vi "Send Temperature Status.vi"(8 "error in (no error)":errorcluster, 11 "Stream in":refnum<class "Stream.lvclass">) -> (0 "error out":errorcluster, 3 "Stream out":refnum<class "Stream.lvclass">)   [LabVIEW 2018, in "Stream.lvclass"]
uses:
  Stream.lvclass
  Stream.lvclass/Stream.ctl
  Interface/Interface.lvclass/Interface.ctl
  Interface/Interface.lvclass
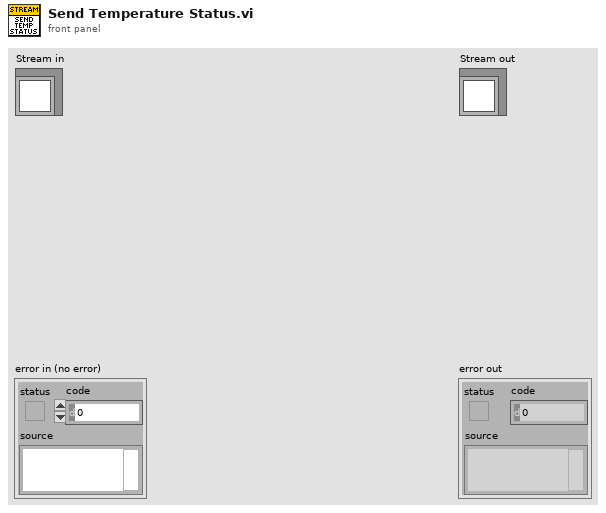
[diagram p1: front panel]
types:
  T1 = cluster{"Current Temperature":i16, "Temperatue Status":string}
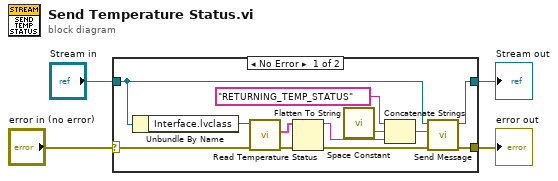
[diagram p0: block diagram]
diagram:
  n1 = case shown="No Error" "error in (no error)" {
    selector: "error in (no error)" -> [w7 w18]
    tunnel: [w16 w18] -> w2
    tunnel: [w14 w17] -> w1
    tunnel: "Stream in" -> [w15 w17]
    frame No Error {
      n2 = Unbundle By Name(w15) -> ("Interface.lvclass"=w6:refnum<class "Interface.lvclass">)
      n3 = call "Read Temperature Status.vi"("error in (no error)"=w7, "Interface in"=w6) -> ("error out"=w8:errorcluster, "Temperature Status"=w5:T1)  [unwired: 7 in, 1 out]
      n4 = Flatten To String(anything=w5, error in (no error)=w8) -> (data string=w10:string, error out=w13:errorcluster)  [unwired: 2 in, 1 out]
      n5 = call <vilib>:"Space Constant.vi"() -> ("String"=w11:string)
      n6 = Concatenate Strings("RETURNING_TEMP_STATUS", w11, w10) -> (w9:string)
      n7 = call "Send Message.vi"("error in (no error)"=w13, "Message"=w9, "Stream in"=w15) -> ("error out"=w16:errorcluster, "Stream out"=w14:refnum<class "Stream.lvclass">)  [unwired: 7 in]
    }
    frame Error {
    }
  }
  "error out" <- w2
  "Stream out" <- w1
